vi "Newmark-GotoOne.vi"(0 "Table VRN IN":refnum<visa-resource-name>="COM9", 2 "Bool Refnum":refnum<vi>, 5 "StageTAG":string, 9 "Notify?":bool, 11 "Error IN":errorcluster, 13 "Position":dbl) -> (4 "Table VRN OUT":refnum<visa-resource-name>="COM9", 15 "Error OUT":errorcluster)   [LabVIEW 2011]
uses:
  Comm/SerialCommError.vi
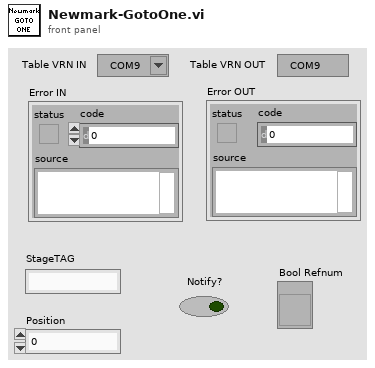
[diagram p1: front panel]
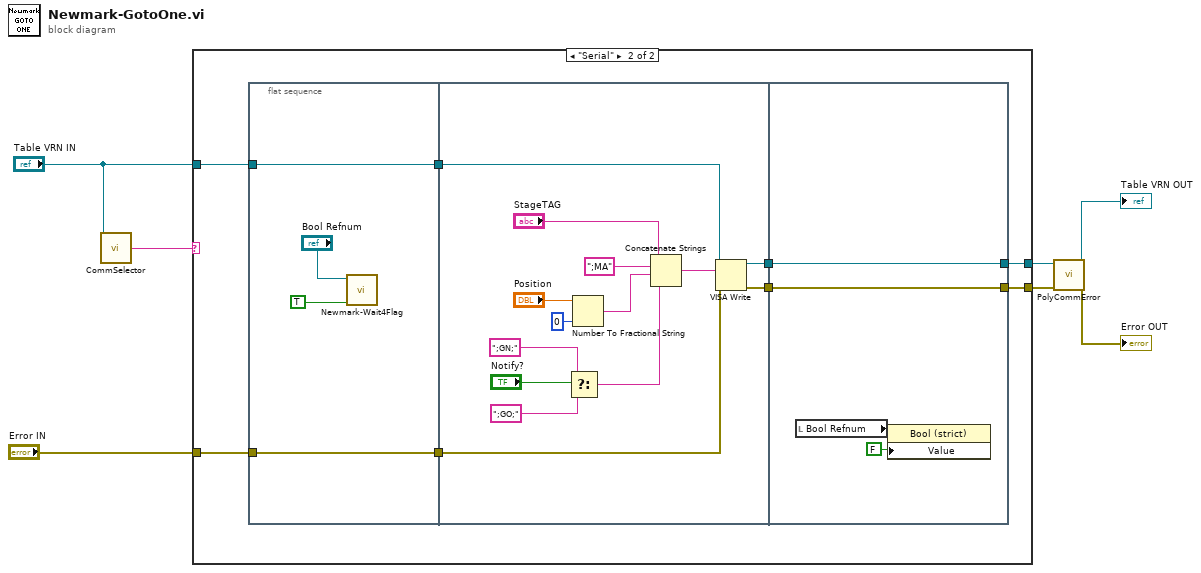
[diagram p0: block diagram]
diagram:
  n1 = call "CommSelector.vi"("VISA resource name"="Table VRN IN") -> ("CommType"=w7:string)  [unwired: 13 in, 1 out]
  n2 = case shown="\"Serial\"" w7 {
    tunnel: "Table VRN IN" -> [w9 w16]
    tunnel: "Error IN" -> [w8 w14]
    tunnel: [w9 w13] -> w2
    tunnel: [w8 w11] -> w1
    frame "Unknown", Default {
    }
    frame "Serial" {
      n3 = flat-sequence {
        tunnel: [w19] -> w17
        tunnel: w16 -> [w19]
        tunnel: [w18] -> w15
        tunnel: w14 -> [w18]
        tunnel: w17 -> [w25]
        tunnel: w15 -> [w24]
        tunnel: [w23] -> w12
        tunnel: [w22] -> w10
        tunnel: [w37] -> w13
        tunnel: w12 -> [w37]
        tunnel: [w36] -> w11
        tunnel: w10 -> [w36]
        frame #0 {
          n4 = call "Newmark-Wait4Flag.vi"("Raise Flag ?"=TRUE, "Ctl Refnum IN"="Bool Refnum") -> ()  [unwired: 8 in, 2 out]
        }
        frame #1 {
          n5 = Select(t=";GN;" ("string"), s="Notify?", f=";GO;" ("string")) -> (s? t:f=w28:string)
          n6 = Number To Fractional String(number="Position", precision (6)=i16 0) -> (F-format string=w31:string)  [unwired: 2 in]
          n7 = Concatenate Strings("StageTAG", ";MA" ("string"), w31, w28) -> (w33:string)
          n8 = VISA Write(VISA resource name=w25, write buffer=w33, error in (no error)=w24) -> (VISA resource name out=w23:refnum<visa-resource-name>, error out=w22:errorcluster)  [unwired: 1 out]
        }
        frame #2 {
          n9 = local read "Bool Refnum"() -> (w39:refnum<vi>)
          n10 = property class="Bool (strict)"(reference=w39, "Value"=FALSE) -> ()  [unwired: 1 in, 2 out]
        }
      }
    }
  }
  n11 = call-poly "PolyCommError.vi"("VISA IN"=w2, "error IN"=w1) -> ("VISA OUT"=→"Table VRN OUT":refnum<visa-resource-name>, "error OUT"=→"Error OUT":errorcluster)  [unwired: 11 in, 1 out]
